vi "createClassDataAndVersionsLUT.vi"(8 "error in (no error)":errorcluster, 9 "allClassNames":string[](array[string]), 10 "classHierarchyLUT":variant) -> (0 "error out":errorcluster, 1 "classPrivateDataLUT":variant, 2 "classVersionNumbersLUT":variant, 4 "classPrivateDataLabelLUT":variant)   [LabVIEW 2020, in "openg_variant.lvlib" / "Reflection.lvclass"]
doc: "GCraftsman JSON Object Serialization Toolkit\nwww.GCraftsman.com\nCopyright (c) 2017, GCraftsman"
uses:
  Reflection.lvclass
  Reflection.lvclass/Reflection.ctl
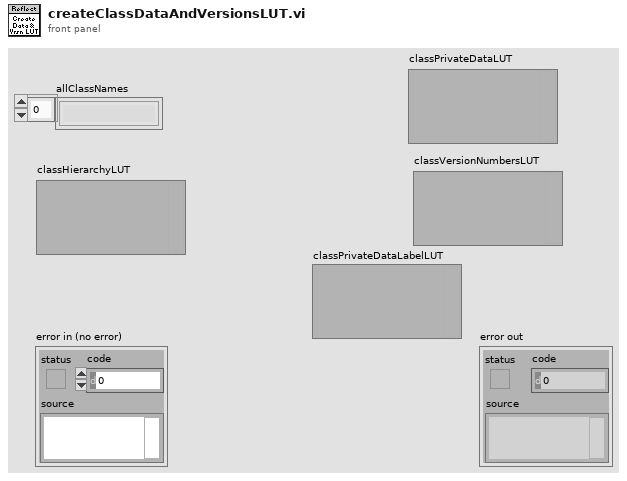
[diagram p1: front panel]
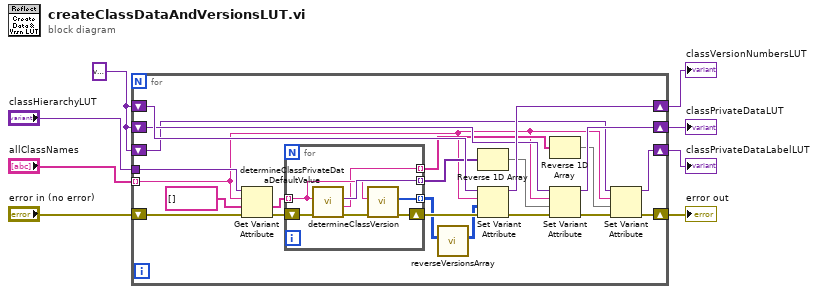
[diagram p0: block diagram]
diagram:
  w2 = variant ("classHierarchyLUT")
  n1 = for {
    tunnel: "allClassNames" -> [w16] mode=indexing
    shift-right: [w26] -> w6
    shift-left: w2 -> [w27]
    shift-right: [w24] -> w5
    shift-left: w2 -> [w25]
    shift-right: [w14] -> w3
    shift-left: "error in (no error)" -> [w20]
    tunnel: "classHierarchyLUT" -> [w29]
    shift-right: [w12] -> w1
    shift-left: w2 -> [w13]
    n2 = Get Variant Attribute(Variant=w29, name=w16, default value (empty Variant)=string[] [] ("classHierarchy"), error in=w20) -> (value=w28:string[], error out=w23:errorcluster)  [unwired: 2 out]
    n3 = for {
      tunnel: w28 -> [w35] mode=indexing
      tunnel: [w36] -> w19 mode=indexing
      tunnel: [w34] -> w9 mode=indexing
      shift-right: [w32] -> w22
      shift-left: w23 -> [w33]
      tunnel: [w31] -> w18 mode=indexing
      n4 = call "determineClassPrivateDataDefaultValue.vi"("error in (no error)"=w33, "className"=w35) -> ("error out"=w37:errorcluster, "privateDataClusterLabel"=w31:string, "privateDataDefaultValue"=w36:variant)  [unwired: 7 in]
      n5 = call "determineClassVersion.vi"("error in (no error)"=w37, "className"=w35) -> ("error out"=w32:errorcluster, "versionNumber"=w34:u8[])  [unwired: 8 in]
    }
    n6 = call "reverseVersionsArray.vi"("versionsArray"=w9) -> ("reversedVersionsArray"=w10:u8[][])  [unwired: 10 in]
    n7 = Reverse 1D Array(array=w19) -> (reversed array=w11:variant[])
    n8 = Set Variant Attribute(Variant=w27, name=w16, value=w10, error in=w22) -> (Variant out=w26:variant, error out=w21:errorcluster)  [unwired: 1 out]
    n9 = Reverse 1D Array(array=w18) -> (reversed array=w17:string[])
    n10 = Set Variant Attribute(Variant=w25, name=w16, value=w11, error in=w21) -> (Variant out=w24:variant, error out=w15:errorcluster)  [unwired: 1 out]
    n11 = Set Variant Attribute(Variant=w13, name=w16, value=w17, error in=w15) -> (Variant out=w12:variant, error out=w14:errorcluster)  [unwired: 1 out]
  }
  "error out" <- w3
  "classVersionNumbersLUT" <- w6
  "classPrivateDataLUT" <- w5
  "classPrivateDataLabelLUT" <- w1
